vi "P4CMD File History.vi"(6 "versions":string[](array[string]), 7 "advanced options":variant, 8 "error in (no error)":errorcluster, 10 "files":path[](array[path]), 11 "source control reference in":T1) -> (0 "error out":errorcluster, 2 "status message":string, 3 "source control reference out":T1, 5 "file changed?":bool)   [LabVIEW 2020, in "NI_SCC_P4CMD.lvlib"]
uses:
  <vilib>/SourceControl/Providers/P4CMD/NI_SCC_P4CMD.lvlib
  <vilib>/SourceControl/sccapi/SCCAPI Refnum.ctl
  <vilib>/SourceControl/Providers/P4CMD/P4CMD Operations.ctl
  <vilib>/SourceControl/Providers/P4CMD/P4CMD Mgr Functions.ctl
  <vilib>/SourceControl/support/SCCSup Message Strings GLBL.vi
  <vilib>/SourceControl/sccapi/NI_SCC.lvlib
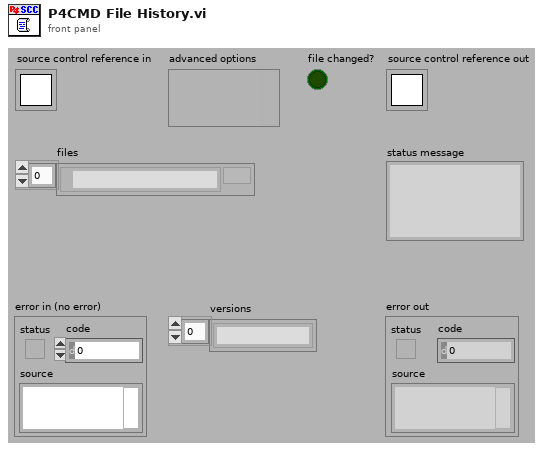
[diagram p1: front panel]
types:
  T1 = typedef "NI_SCC.lvlib/SCCAPI Refnum.ctl" = refnum<k1>
  T2 = typedef "NI_SCC_P4CMD.lvlib/P4CMD Mgr Functions.ctl" = enum16{"Init", "Open", "Set Config Opts", "Initialized?", "IsRefValid?", "Get Config Opts", "Get Global Commands", "Close", "Uninit"}
  T3 = typedef "NI_SCC_P4CMD.lvlib/P4CMD Operations.ctl" = enum16{"get all clients", "get all users", "describe changelist", "sync from depot", "open for edit", "submit to depot", "revert", "add to depot", "remove from depot", "print files revisions", "compare client file", "print depot file contents", "list opened files", "get file info", "lock files", "edit changelist spec", "info", "set variables"}
  T4 = typedef "NI_SCC_P4CMD.lvlib/P4CMD SCC File Status.ctl" = cluster{"source controlled":bool, "open by user":bool, "open by other":bool, "out of date":bool, "deleted":bool, "locked by user":bool, "locked by other":bool, "open for add by user":bool, "open for delete by user":bool}
  T5 = typedef "NI_SCC_P4CMD.lvlib/P4CMD Advanced Options.ctl" = cluster{"lock files?":bool, "suppress dialogs?":bool}
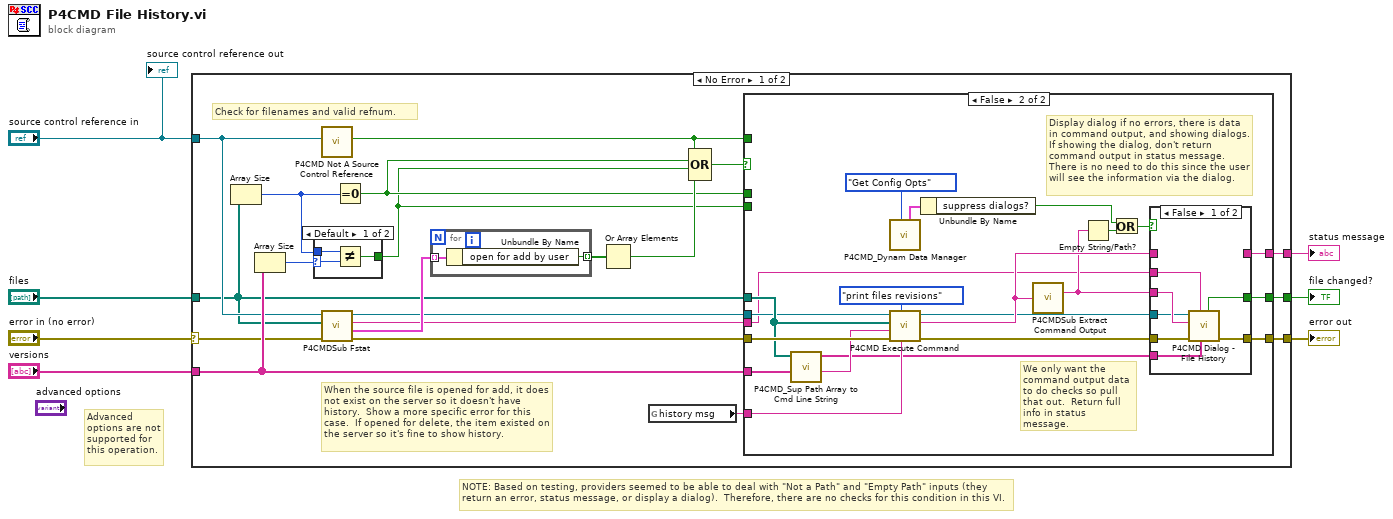
[diagram p0: block diagram]
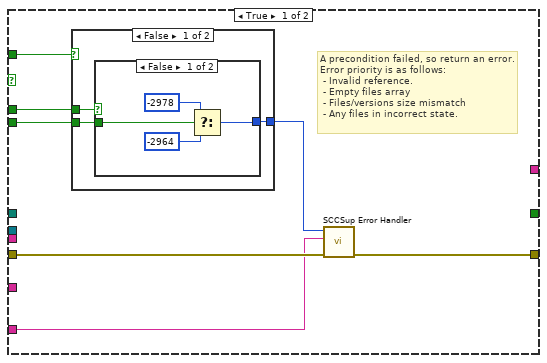
[diagram p3: hidden frame]
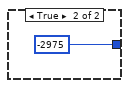
[diagram p4: hidden frame]
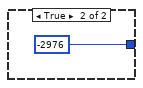
[diagram p5: hidden frame]
diagram:
  # "Advanced options are not supported for this operation."
  # "NOTE: Based on testing, providers seemed to be able to deal with \"Not a Path\" and \"Empty Path\" inputs (they return an error, status message, or display a dialog).  Therefore, there are no checks for this condition in this VI."
  n1 = case shown="No Error" "error in (no error)" {
    selector: "error in (no error)" -> [w18 w79]
    tunnel: [w22 w79] -> w6
    tunnel: "source control reference in" -> [w15 _]
    tunnel: [w27 _] -> w4
    tunnel: "files" -> [w13 _]
    tunnel: [w24 _] -> w2
    tunnel: "versions" -> [w21 _]
    frame No Error {
      # "When the source file is opened for add, it does not exist on the server so it doesn't have history.  Show a more specific error for this case.  If opened for delete, the item existed on the server so it's fine to show history."
      # "Check for filenames and valid refnum."
      n2 = Array Size(array=w13) -> (size(s)=w19:i32)
      n3 = Array Size(array=w21) -> (size(s)=w20:i32)
      n4 = case shown="Default" w20 {
        selector: w20 -> [w30 _]
        tunnel: [w32 _] -> w9
        tunnel: w19 -> [w31 _]
        frame Default {
          n5 = Not Equal?(x=w31, y=w30) -> (x != y?=w32:bool)
        }
        frame 0 {
        }
      }
      n6 = call <vilib>:"P4CMD Not A Source Control Reference.vi"("source control reference in"=w15) -> ("not a source control reference?"=w25:bool)  [unwired: 9 in, 1 out]
      n7 = call <vilib>:"P4CMDSub Fstat.vi"("error in (no error)"=w18, "files"=w13, "source control reference in"=w15) -> ("error out"=w17:errorcluster, "files status"=w16:T4[], "fstat output"=w8:string, "source control reference out"=w14:T1)  [unwired: 5 in]
      n8 = Equal To 0?(x=w19) -> (x = 0?=w10:bool)
      n9 = for {
        tunnel: w16 -> [w29] mode=indexing
        tunnel: [w28] -> w12 mode=indexing
        n10 = Unbundle By Name(w29) -> ("open for add by user"=w28:bool)
      }
      n11 = Or Array Elements(Boolean array=w12) -> (logical OR=w11:bool)
      n12 = global read "SCCSup Message Strings GLBL.vi" "history msg"() -> (w23:string)
      n13 = Compound Arithmetic op=OR(w25, w10, w9, w11) -> (w26:bool)
      n14 = case shown="False" w26 {
        tunnel: [_ w57] -> w27
        tunnel: w13 -> [_ w65]
        tunnel: w25 -> [w39 _]
        tunnel: [_ w53] -> w24
        tunnel: w17 -> [w37 w67]
        tunnel: [w36 w62] -> w22
        tunnel: w21 -> [_ w69]
        tunnel: w10 -> [w38 _]
        tunnel: w23 -> [w34 w64]
        tunnel: w14 -> [_ w56]
        tunnel: w9 -> [w33 _]
        tunnel: w8 -> [_ w49]
        frame True {
          # "A precondition failed, so return an error. \nError priority is as follows:\n - Invalid reference.  \n - Empty files array\n - Files/versions size mismatch\n - Any files in incorrect state."
          n15 = case shown="False" w39 {
            tunnel: [w42 -2976 ("result")] -> w35
            tunnel: w38 -> [w40 _]
            tunnel: w33 -> [w41 _]
            frame False {
              n16 = case shown="False" w40 {
                tunnel: [w44 -2975 ("result")] -> w42
                tunnel: w41 -> [w43 _]
                frame False {
                  n17 = Select(t=-2978 ("result"), s=w43, f=-2964 ("result")) -> (s? t:f=w44:i32)
                }
                frame True {
                }
              }
            }
            frame True {
            }
          }
          n18 = call <vilib>:"SCCSup Error Handler.vi"("error in (no error)"=w37, "operation message"=w34, "scc error code"=w35) -> ("error out"=w36:errorcluster)  [unwired: 8 in]
        }
        frame False {
          # "We only want the command output data to do checks so pull that out.  Return full info in status message."
          # "Display dialog if no errors, there is data in command output, and showing dialogs.\nIf showing the dialog, don't return command output in status message.  There is no need to do this since the user will see the information via the dialog."
          n19 = call <vilib>:"P4CMD_Sup Path Array to Cmd Line String.vi"("modifiers"=w69, "files"=w65) -> ("string output"=w66:string, "converted file strings"=w61:string[])  [unwired: 8 in]
          n20 = call <vilib>:"P4CMD_Dynam Data Manager.vi"("function"=P4CMD_Mgr_Functions."Get Config Opts") -> ("adv cfg options out"=w59:T5)  [unwired: 5 in, 5 out]
          n21 = call <vilib>:"P4CMD Execute Command.vi"("operation message"=w64, "p4 operation"=P4CMD_Operations."print files revisions", "error in (no error)"=w67, "input string"=w66, "files"=w65, "source control reference in"=w56) -> ("error out"=w63:errorcluster, "command information"=w55:string, "source control reference out"=w52:T1)  [unwired: 3 in]
          n22 = Unbundle By Name(w59) -> ("suppress dialogs?"=w50:bool)
          n23 = call <vilib>:"P4CMDSub Extract Command Output.vi"("bundled message"=w55) -> ("command output"=w54:string)  [unwired: 13 in, 1 out]
          n24 = Empty String/Path?(string/path=w54) -> (empty?=w51:bool)
          n25 = Or(x=w50, y=w51) -> (x .or. y?=w58:bool)
          n26 = case shown="False" w58 {
            tunnel: w54 -> [w74 _]
            tunnel: w63 -> [w76 w78]
            tunnel: [w75 w78] -> w62
            tunnel: w61 -> [w73 _]
            tunnel: w55 -> [_ w77]
            tunnel: [_ w77] -> w57
            tunnel: [w72 _] -> w53
            tunnel: w52 -> [w71 _]
            tunnel: w49 -> [w70 _]
            frame False {
              n27 = call <vilib>:"P4CMD Dialog - File History.vi"("files"=w73, "fstat info"=w70, "error in (no error)"=w76, "revision string"=w74, "source control reference in"=w71) -> ("error out"=w75:errorcluster, "file changed?"=w72:bool)  [unwired: 5 in]
            }
            frame True {
            }
          }
        }
      }
    }
    frame Error {
    }
  }
  "error out" <- w6
  "status message" <- w4
  "file changed?" <- w2
  "source control reference out" <- "source control reference in"
